vi "运维调试.vi"() -> ()   [LabVIEW 2016]
uses:
  <vilib>/Utility/miscctls.llb/LVPointTypeDef.ctl
  PLC/PLC.lvlib
  <vilib>/Utility/config.llb/NI_LVConfig.lvlib
panel:
  in  "运维调试菜单":T1(xcontrol)
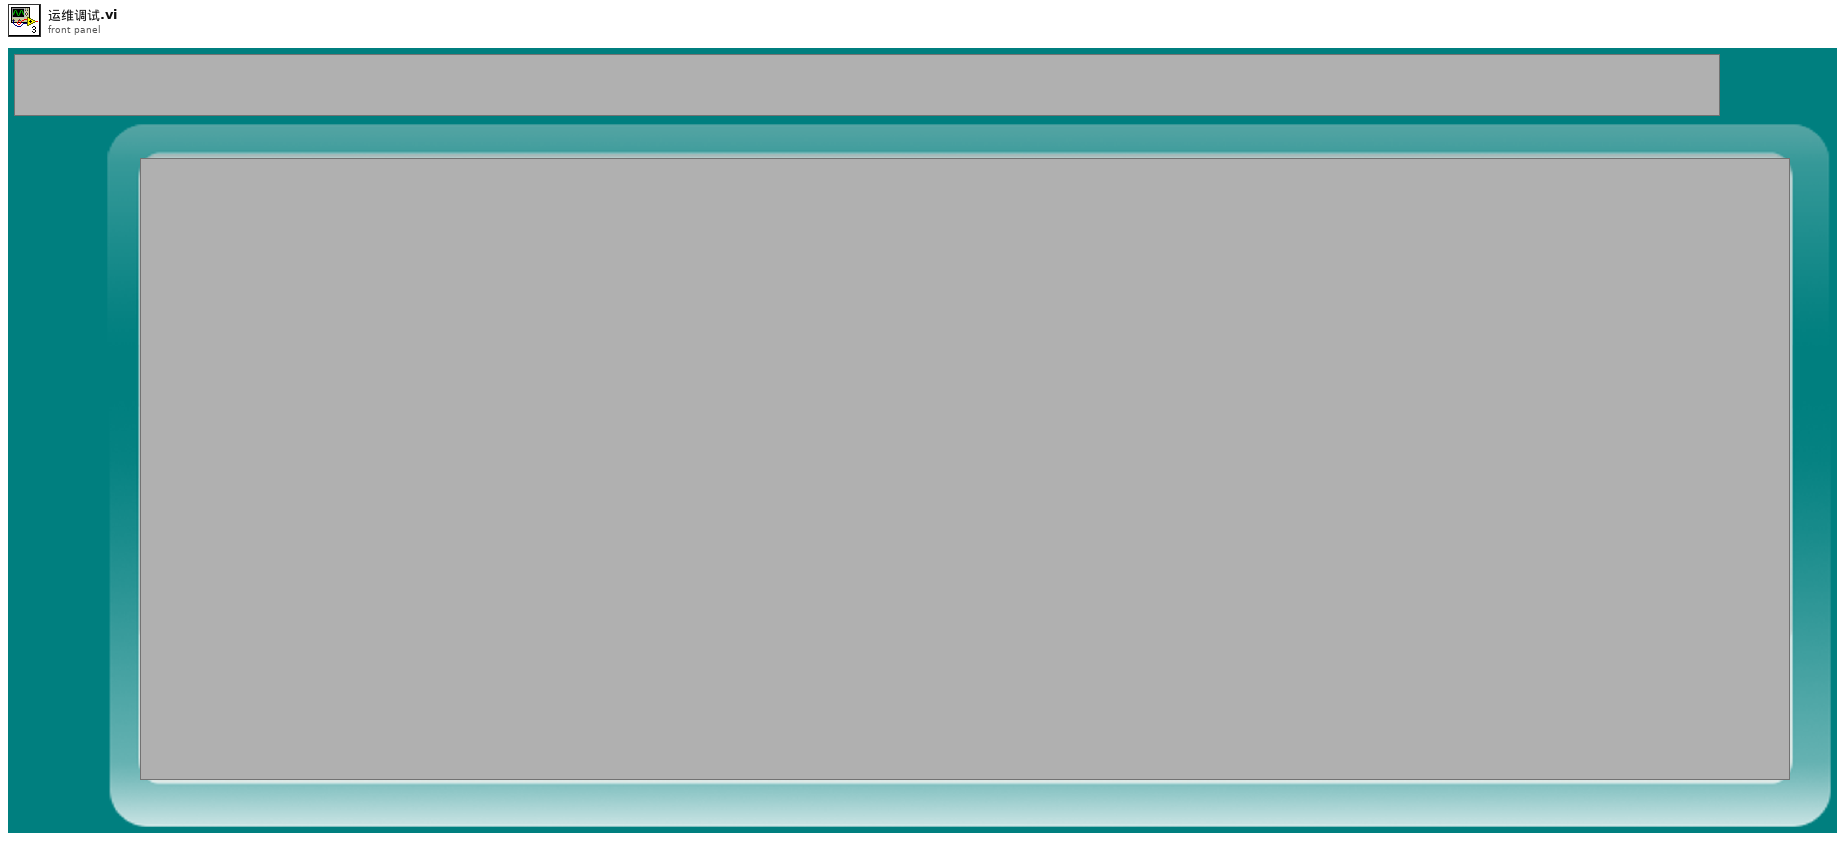
[diagram p1: front panel]
types:
  T1 = enum16{"电源管理", "采配水", "氨氮", "总磷总氮", "多参数", "CODMn", "CODcr", "流量计", "质控单元", "超标留样", "其他"}
  T2 = typedef "NI_LVConfig.lvlib/Config Data RefNum.ctl" = refnum<k1>
  T3 = typedef "LVPointTypeDef.ctl" = cluster{"Horizontal":i16, "Vertical":i16}
  T4 = enum16{"Enabled", "Disabled", "Disabled and Grayed Out"}
  T5 = enum32{"Bad", "Idle", "Run top level", "Running"}
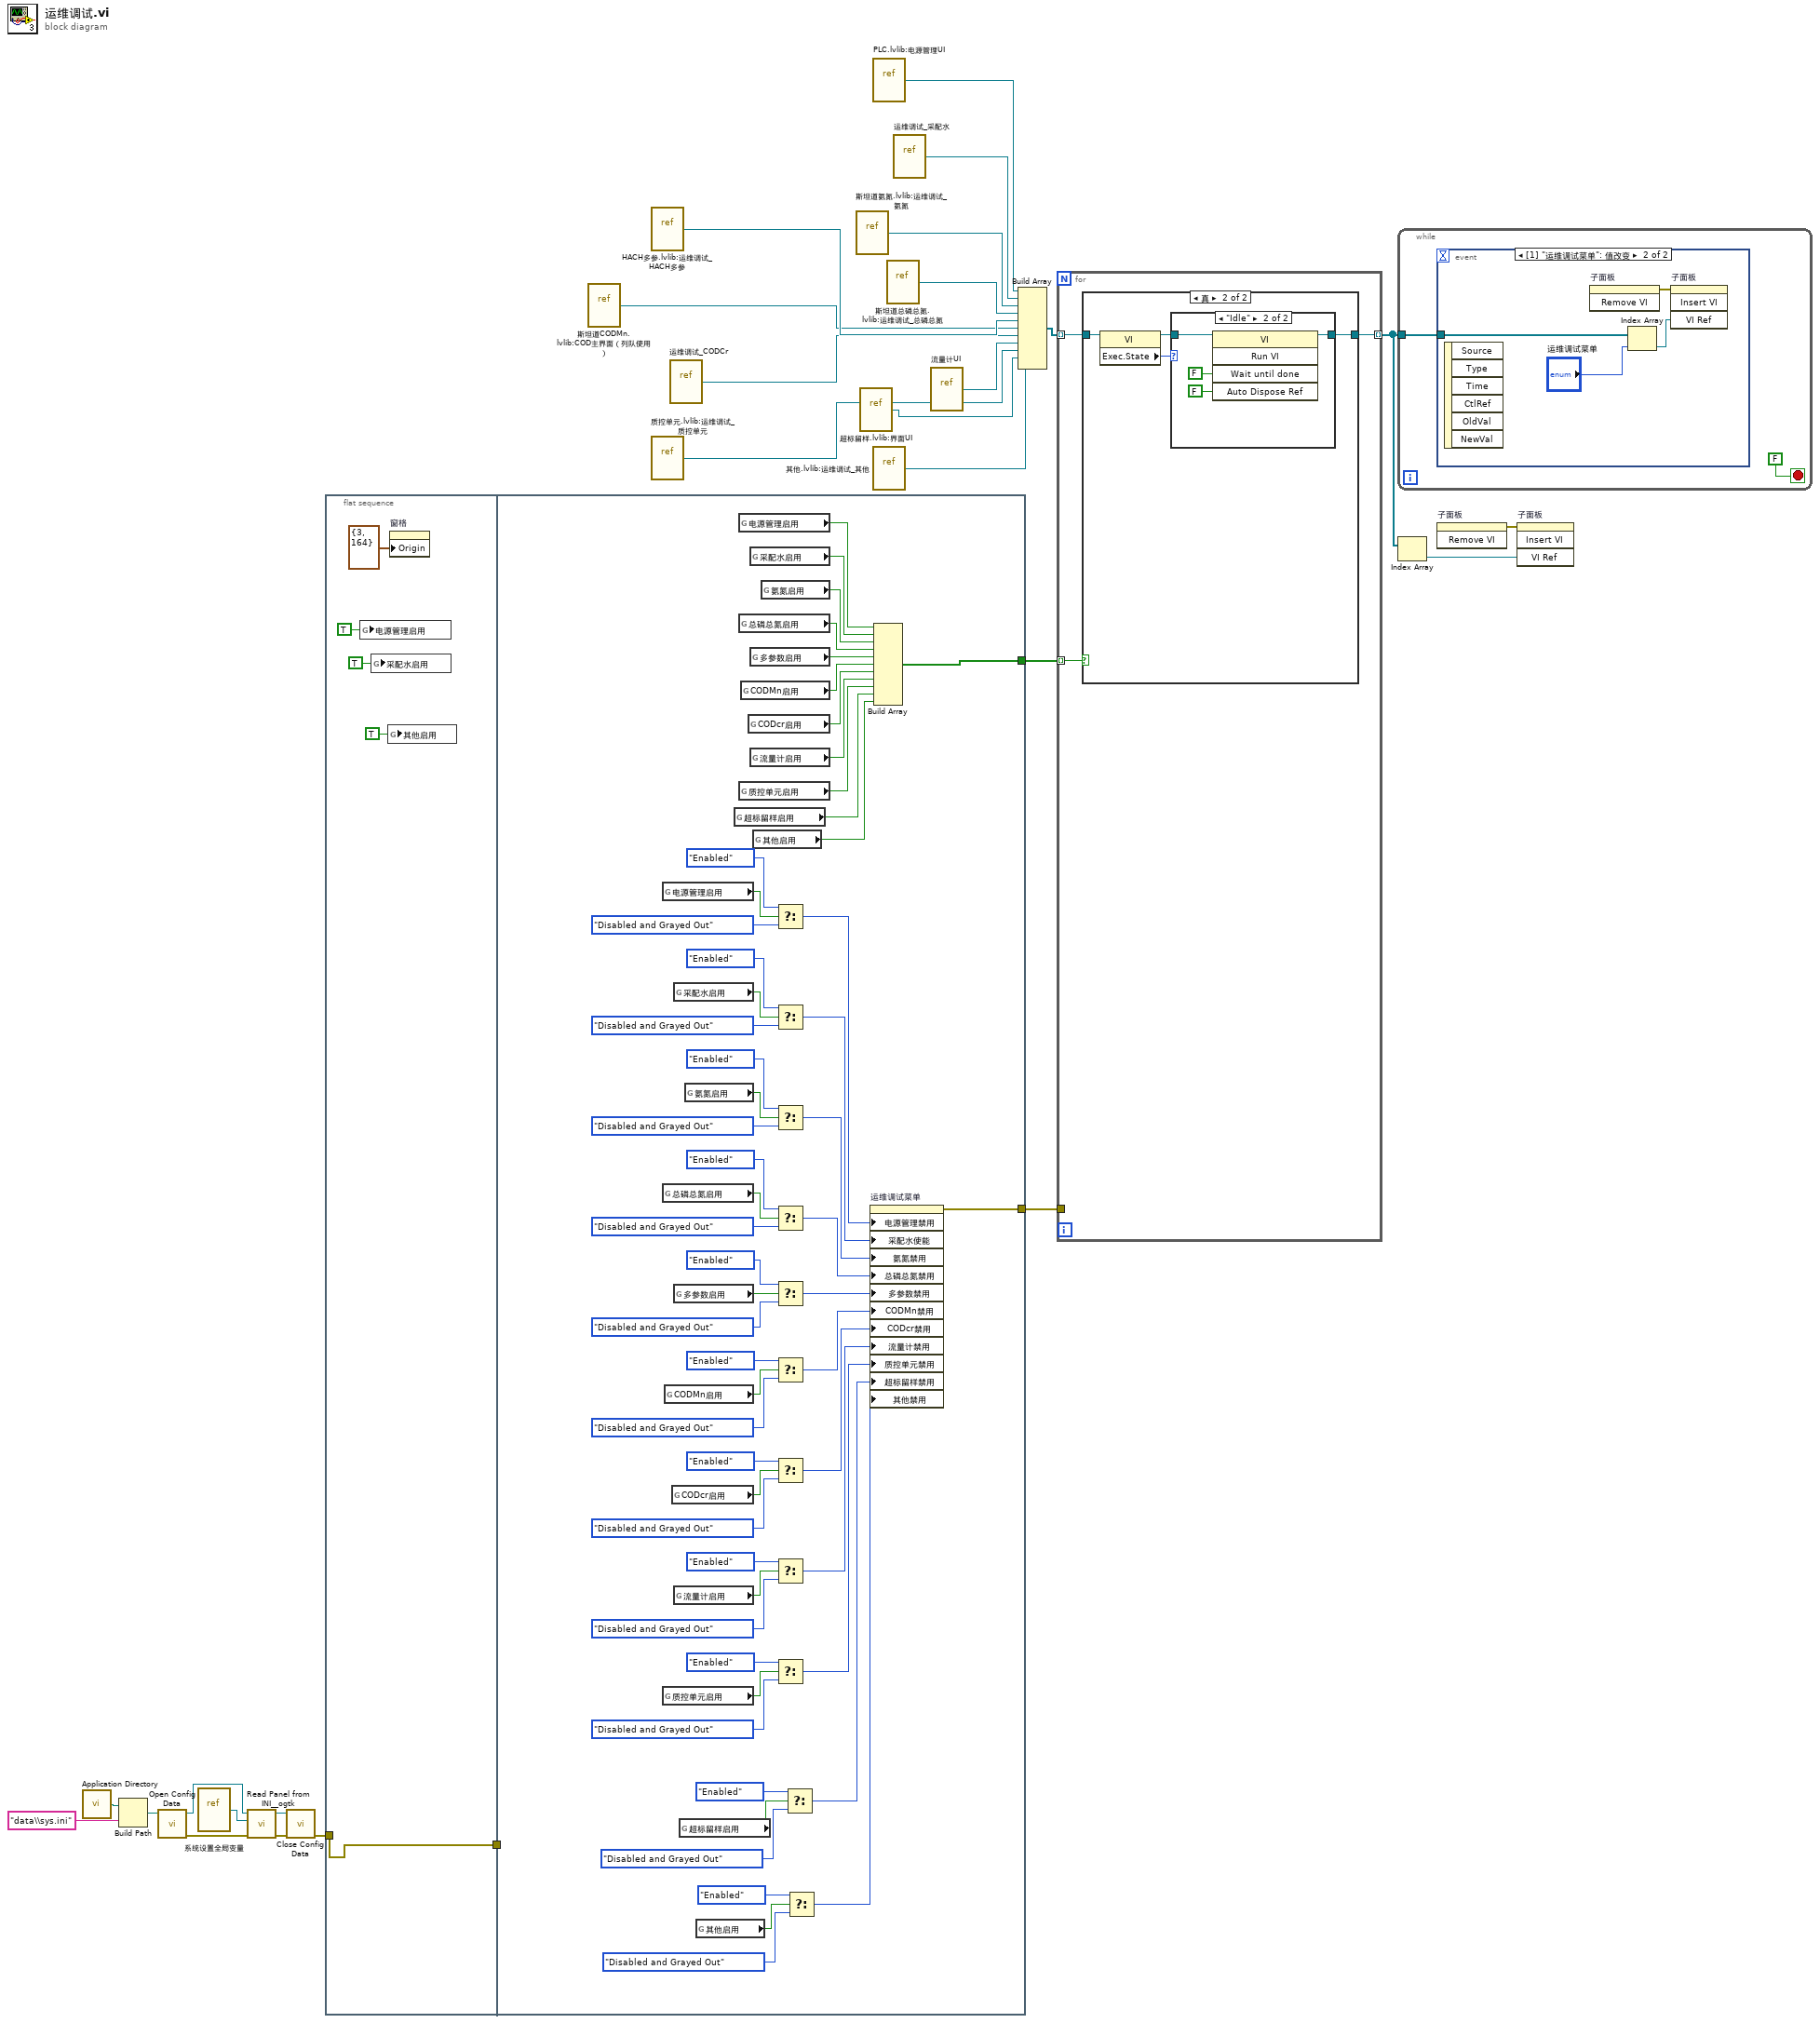
[diagram p0: block diagram]
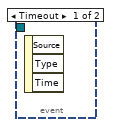
[diagram p4: hidden frame]
diagram:
  n1 = call <vilib>:"Application Directory.vi"() -> ("Application Directory"=w6:path)
  n2 = Build Path(base path=w6, name or relative path="data\\sys.ini" ("名称或相对路径")) -> (appended path=w4:path)
  n3 = call <vilib>:"Open Config Data.vi"("configuration file path"=w4) -> ("error out"=w13:errorcluster, "refnum"=w12:T2)  [unwired: 8 in, 1 out]
  n4 = vi-ref "系统设置全局变量.vi"() -> (w11:refnum<vi>)
  n5 = call <userlib>:"Read Panel from INI__ogtk.vi"("error in (no error)"=w13, "VI ref"=w11, "refnum"=w12) -> ("error out"=w10:errorcluster, "refnum out"=w9:T2)  [unwired: 7 in]
  n6 = call <vilib>:"Close Config Data.vi"("error in (no error)"=w10, "refnum"=w9) -> ("error out"=w8:errorcluster)  [unwired: 8 in, 1 out]
  n7 = flat-sequence {
    tunnel: w8 -> [w32]
    tunnel: [w32] -> w7
    tunnel: [w70] -> w14
    tunnel: w7 -> [_]
    tunnel: [w60] -> w3
    frame #0 {
      n8 = global write "系统设置全局变量.vi" "电源管理启用"(TRUE ("电源管理启用")) -> ()
      n9 = global write "系统设置全局变量.vi" "采配水启用"(TRUE ("采配水启用")) -> ()
      n10 = global write "系统设置全局变量.vi" "其他启用"(TRUE ("其他启用")) -> ()
      n11 = property on="窗格" class="Pane"("Origin"=T3 {"Horizontal"=3, "Vertical"=164} ("原点")) -> ()  [unwired: 2 in, 2 out]
    }
    frame #1 {
      n12 = global read "系统设置全局变量.vi" "电源管理启用"() -> (w89:bool)
      n13 = global read "系统设置全局变量.vi" "总磷总氮启用"() -> (w83:bool)
      n14 = global read "系统设置全局变量.vi" "质控单元启用"() -> (w76:bool)
      n15 = global read "系统设置全局变量.vi" "CODMn启用"() -> (w79:bool)
      n16 = global read "系统设置全局变量.vi" "CODcr启用"() -> (w78:bool)
      n17 = global read "系统设置全局变量.vi" "采配水启用"() -> (w86:bool)
      n18 = global read "系统设置全局变量.vi" "多参数启用"() -> (w81:bool)
      n19 = global read "系统设置全局变量.vi" "流量计启用"() -> (w77:bool)
      n20 = global read "系统设置全局变量.vi" "超标留样启用"() -> (w34:bool)
      n21 = global read "系统设置全局变量.vi" "氨氮启用"() -> (w85:bool)
      n22 = global read "系统设置全局变量.vi" "其他启用"() -> (w75:bool)
      n23 = global read "系统设置全局变量.vi" "超标留样启用"() -> (w39:bool)
      n24 = global read "系统设置全局变量.vi" "电源管理启用"() -> (w61:bool)
      n25 = global read "系统设置全局变量.vi" "总磷总氮启用"() -> (w64:bool)
      n26 = global read "系统设置全局变量.vi" "质控单元启用"() -> (w69:bool)
      n27 = global read "系统设置全局变量.vi" "CODMn启用"() -> (w66:bool)
      n28 = global read "系统设置全局变量.vi" "CODcr启用"() -> (w67:bool)
      n29 = global read "系统设置全局变量.vi" "采配水启用"() -> (w62:bool)
      n30 = global read "系统设置全局变量.vi" "多参数启用"() -> (w65:bool)
      n31 = global read "系统设置全局变量.vi" "流量计启用"() -> (w68:bool)
      n32 = global read "系统设置全局变量.vi" "其他启用"() -> (w38:bool)
      n33 = global read "系统设置全局变量.vi" "氨氮启用"() -> (w63:bool)
      n34 = Select(t=T4."Enabled" ("电源管理禁用"), s=w89, f=T4."Disabled and Grayed Out" ("电源管理禁用")) -> (s? t:f=w88:T4)
      n35 = Select(t=T4."Enabled" ("电源管理禁用"), s=w86, f=T4."Disabled and Grayed Out" ("电源管理禁用")) -> (s? t:f=w87:T4)
      n36 = Select(t=T4."Enabled" ("电源管理禁用"), s=w85, f=T4."Disabled and Grayed Out" ("电源管理禁用")) -> (s? t:f=w84:T4)
      n37 = Select(t=T4."Enabled" ("电源管理禁用"), s=w83, f=T4."Disabled and Grayed Out" ("电源管理禁用")) -> (s? t:f=w82:T4)
      n38 = Select(t=T4."Enabled" ("电源管理禁用"), s=w81, f=T4."Disabled and Grayed Out" ("电源管理禁用")) -> (s? t:f=w80:T4)
      n39 = Select(t=T4."Enabled" ("电源管理禁用"), s=w79, f=T4."Disabled and Grayed Out" ("电源管理禁用")) -> (s? t:f=w74:T4)
      n40 = Select(t=T4."Enabled" ("电源管理禁用"), s=w78, f=T4."Disabled and Grayed Out" ("电源管理禁用")) -> (s? t:f=w73:T4)
      n41 = Select(t=T4."Enabled" ("电源管理禁用"), s=w77, f=T4."Disabled and Grayed Out" ("电源管理禁用")) -> (s? t:f=w72:T4)
      n42 = Select(t=T4."Enabled" ("电源管理禁用"), s=w76, f=T4."Disabled and Grayed Out" ("电源管理禁用")) -> (s? t:f=w71:T4)
      n43 = Select(t=T4."Enabled" ("电源管理禁用"), s=w34, f=T4."Disabled and Grayed Out" ("电源管理禁用")) -> (s? t:f=w33:T4)
      n44 = Select(t=T4."Enabled" ("电源管理禁用"), s=w75, f=T4."Disabled and Grayed Out" ("电源管理禁用")) -> (s? t:f=w37:T4)
      n45 = property on="运维调试菜单" class="运维调试菜单 (严格)"("电源管理禁用"=w88, "采配水使能"=w87, "氨氮禁用"=w84, "总磷总氮禁用"=w82, "多参数禁用"=w80, "CODMn禁用"=w74, "CODcr禁用"=w73, "流量计禁用"=w72, "质控单元禁用"=w71, "超标留样禁用"=w33, "其他禁用"=w37) -> (error out=w70:errorcluster)  [unwired: 2 in, 1 out]
      n46 = Build Array(w61, w62, w63, w64, w65, w66, w67, w68, w69, w39, w38) -> (w60:bool[])
    }
  }
  n47 = vi-ref "斯坦道CODMn.lvlib:COD主界面（列队使用）.vi"() -> (w19:refnum<vi>)
  n48 = vi-ref "HACH多参.lvlib:运维调试_HACH多参.vi"() -> (w20:refnum<vi>)
  n49 = vi-ref "质控单元.lvlib:运维调试_质控单元.vi"() -> (w17:refnum<vi>)
  n50 = vi-ref "运维调试_CODCr.vi"() -> (w18:refnum<vi>)
  n51 = vi-ref "斯坦道氨氮.lvlib:运维调试_氨氮.vi"() -> (w22:refnum<vi>)
  n52 = vi-ref "超标留样.lvlib:界面UI.vi"() -> (w2:refnum<vi>)
  n53 = vi-ref "PLC.lvlib:电源管理UI.vi"() -> (w16:refnum<vi>)
  n54 = vi-ref "其他.lvlib:运维调试_其他.vi"() -> (w1:refnum<vi>)
  n55 = vi-ref "斯坦道总磷总氮.lvlib:运维调试_总磷总氮.vi"() -> (w21:refnum<vi>)
  n56 = vi-ref "运维调试_采配水.vi"() -> (w23:refnum<vi>)
  n57 = vi-ref "流量计UI.vi"() -> (w15:refnum<vi>)
  n58 = Build Array(w16, w23, w22, w21, w20, w19, w18, w15, w17, w2, w1) -> (w24:refnum<vi>[])
  n59 = for {
    tunnel: w24 -> [w92] mode=indexing
    tunnel: [w91] -> w26 mode=indexing
    tunnel: w3 -> [w90] mode=indexing
    tunnel: w14 -> [_]
    n60 = case shown="真" w90 {
      tunnel: w92 -> [w93 w97]
      tunnel: [w93 w94] -> w91
      frame False {
      }
      frame True {
        n61 = property class="VI"(reference=w97) -> (reference out=w95:refnum<vi>, "Exec.State"=w96:T5)  [unwired: 1 in, 1 out]
        n62 = case shown="\"Idle\"" w96 {
          tunnel: w95 -> [w98 w100]
          tunnel: [w98 w99] -> w94
          frame "Bad", Default {
          }
          frame "Idle" {
            n63 = invoke class="VI" method="Run VI"(reference=w100, "Wait until done"=FALSE ("结束前等待"), "Auto Dispose Ref"=FALSE ("自动销毁引用")) -> (reference out=w99:refnum<vi>)  [unwired: 2 in, 4 out]
          }
        }
      }
    }
  }
  n64 = while {
    tunnel: w26 -> [w103]
    stop <- FALSE stop-if-true
    n65 = event shown="[1] \"运维调试菜单\": 值改变" {
      selector: _ -> [_ _]
      dyn-events: _ -> [_ _]
      timeout: _ -> [_ _]
      tunnel: w103 -> [_ w107]
      event Timeout {
        n66 = event-data() -> ()  [unwired: 1 in, 3 out]
      }
      event "运维调试菜单": Value Change {
        n67 = event-data() -> ()  [unwired: 1 in, 6 out]
        n68 = invoke on="子面板" class="SubPnl" method="Remove VI"() -> (error out=w108:errorcluster)  [unwired: 3 in, 2 out]
        n69 = Index Array(array=w107, index="运维调试菜单") -> (element=w106:refnum<vi>)
        n70 = invoke on="子面板" class="SubPnl" method="Insert VI"(error in=w108, "VI Ref"=w106) -> ()  [unwired: 2 in, 4 out]
      }
    }
  }
  n71 = Index Array(array=w26) -> (element=w25:refnum<vi>)  [unwired: 1 in]
  n72 = invoke on="子面板" class="SubPnl" method="Remove VI"() -> (error out=w27:errorcluster)  [unwired: 3 in, 2 out]
  n73 = invoke on="子面板" class="SubPnl" method="Insert VI"(error in=w27, "VI Ref"=w25) -> ()  [unwired: 2 in, 4 out]
